vi "DypnlIO.vi"(0 "CMDQueue":refnum<queue>) -> ()   [LabVIEW 2019]
uses:
  <vilib>/Utility/miscctls.llb/LVPointTypeDef.ctl
  <vilib>/Utility/miscctls.llb/LVRectTypeDef.ctl
  SubVIs/ControlProperty.ctl
  user32.dll
panel:
  in  "Boolean":bool
  in  "error in (no error)":errorcluster
  out "error out":errorcluster
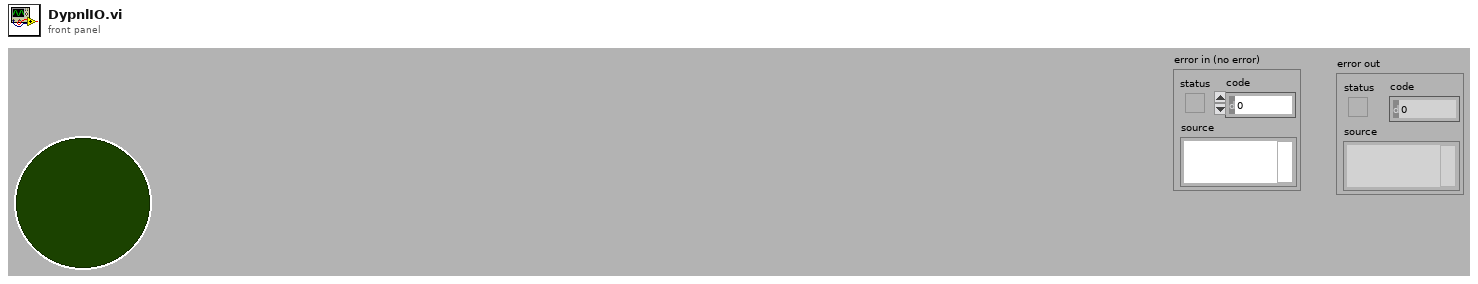
[diagram p1: front panel]
types:
  T1 = enum8{"Enabled", "Disabled", "Disabled and Grayed Out"}
  T2 = typedef "LVPointTypeDef.ctl" = cluster{"Horizontal":i16, "Vertical":i16}
  T3 = typedef "ControlProperty.ctl" = cluster{"Name":string, "WinBounds":T4, "Color":u32, "ShowLabel":bool, "Row/Col":cluster{"Row":u32, "Cols":u32}, "Config":string}
  T4 = typedef "LVRectTypeDef.ctl" = cluster{"Left":i16, "Top":i16, "Right":i16, "Bottom":i16}
  T5 = cluster{"CMD":string, "Parameter":string, "ReturnQueue":refnum<queue>}
  T6 = cluster{"Left":bool, "Top":bool, "Right":bool, "Bottom":bool}
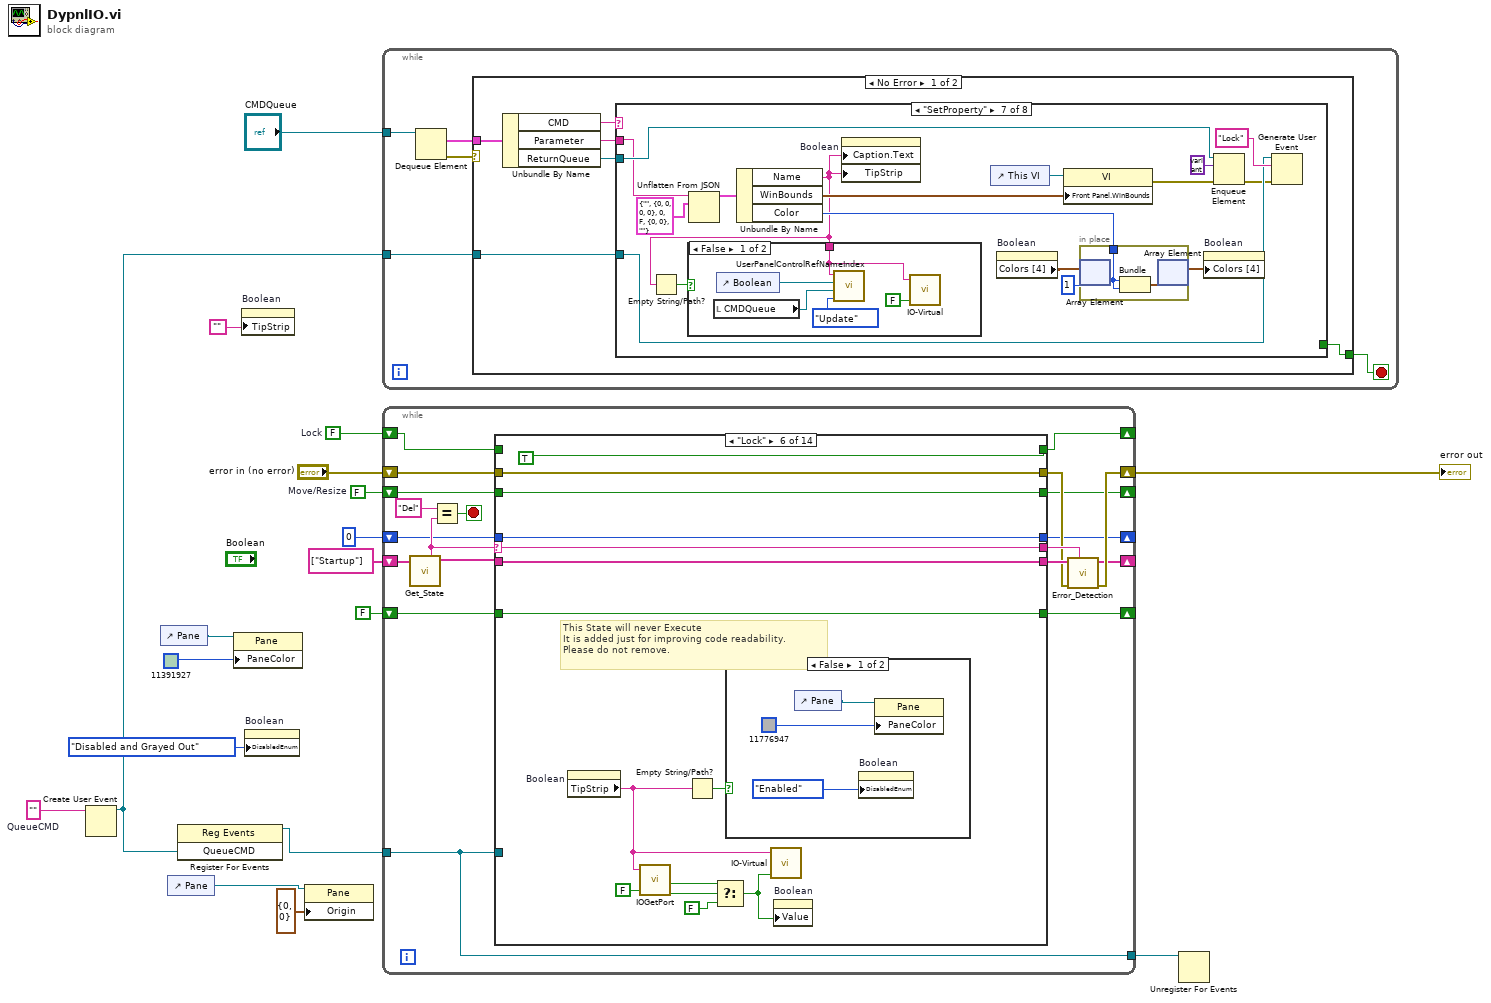
[diagram p0: block diagram]
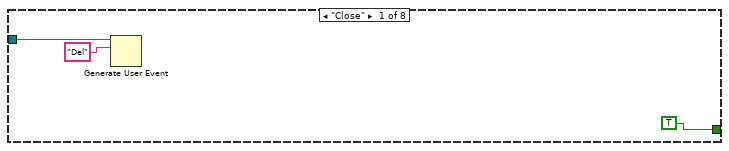
[diagram p2: hidden frame]
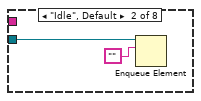
[diagram p3: hidden frame]
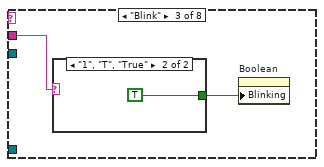
[diagram p4: hidden frame]
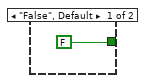
[diagram p5: hidden frame]
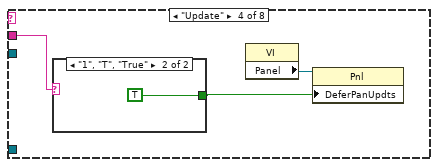
[diagram p6: hidden frame]
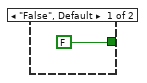
[diagram p7: hidden frame]
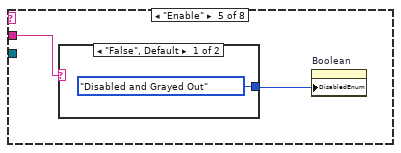
[diagram p8: hidden frame]
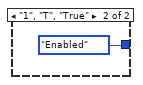
[diagram p9: hidden frame]
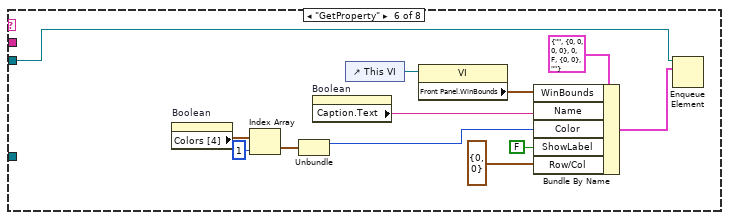
[diagram p10: hidden frame]
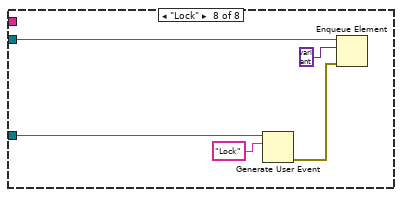
[diagram p12: hidden frame]
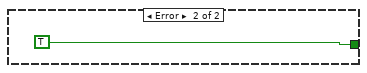
[diagram p13: hidden frame]
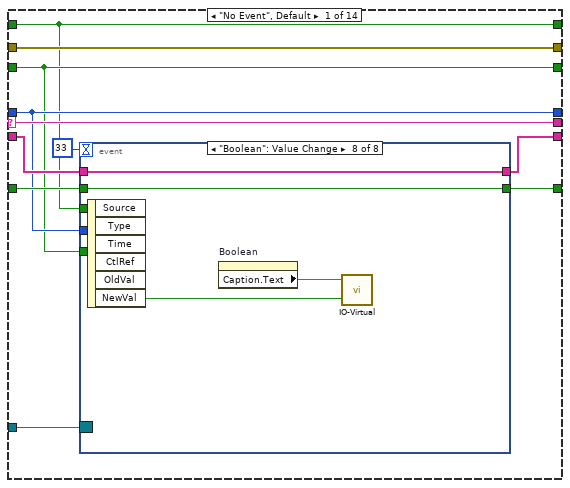
[diagram p14: hidden frame]
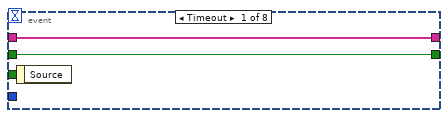
[diagram p15: hidden frame]
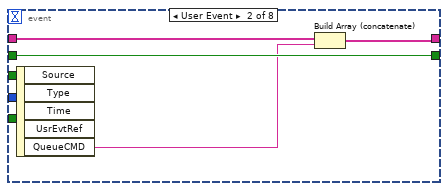
[diagram p16: hidden frame]
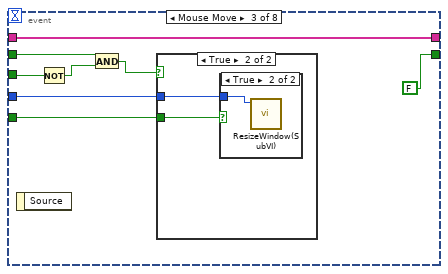
[diagram p17: hidden frame]
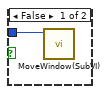
[diagram p19: hidden frame]
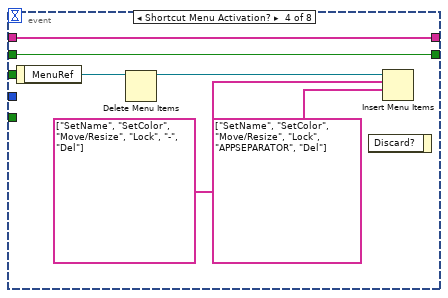
[diagram p20: hidden frame]
diagram:
  w2 = FALSE  # Lock
  w9 = ""  # QueueCMD
  w13 = FALSE  # Move/Resize
  n1 = Create User Event(user event datatype=w9) -> (user event=w6:refnum<user-event>)  [unwired: 1 in, 1 out]
  n2 = control-ref of="Pane"() -> (w4:refnum<vi>)
  n3 = control-ref of="Pane"() -> (w12:refnum<vi>)
  n4 = register-events(w6) -> (reference out=w8:refnum<event-registration>)  [unwired: 2 in, 1 out]
  n5 = property class="Pane"(reference=w4, "PaneColor"=u32 11391927 ("Color Box")) -> ()  [unwired: 1 in, 2 out]
  n6 = property on="Boolean" class="Bool (strict)"("TipStrip"="") -> ()  [unwired: 2 in, 2 out]
  n7 = property on="Boolean" class="Bool (strict)"("DisabledEnum"=T1."Disabled and Grayed Out" ("Disabled")) -> ()  [unwired: 2 in, 2 out]
  n8 = property class="Pane"(reference=w12, "Origin"=T2 {"Horizontal"=0, "Vertical"=0}) -> ()  [unwired: 1 in, 2 out]
  n9 = while {
    tunnel: "CMDQueue" -> [w23]
    tunnel: w6 -> [w19]
    stop <- w21 stop-if-true
    n10 = Dequeue Element(queue=w23) -> (element=w20:T5, error out=w22:errorcluster)  [unwired: 2 in, 2 out]
    n11 = case shown="No Error" w22 {
      tunnel: [w25 TRUE] -> w21
      tunnel: w20 -> [w29 _]
      tunnel: w19 -> [w24 _]
      frame No Error {
        n12 = Unbundle By Name(w29) -> ("CMD"=w28:string, "Parameter"=w26:string, "ReturnQueue"=w27:refnum<queue>)
        n13 = case shown="\"SetProperty\"" w28 {
          tunnel: w27 -> [_ w34 _ _ _ w59 w76 w85]
          tunnel: w26 -> [_ _ w36 w41 w45 _ w71 _]
          tunnel: [TRUE _ _ _ _ _ _ _] -> w25
          tunnel: w24 -> [w31 _ _ _ _ _ w63 w84]
          frame "Close" {
            n14 = Generate User Event(user event=w31, event data cluster="Del" ("event data")) -> ()  [unwired: 2 in, 2 out]
          }
          frame "Idle", Default {
            n15 = Enqueue Element(queue=w34, element="") -> ()  [unwired: 2 in, 3 out]
          }
          frame "Blink" {
            n16 = case shown="\"1\", \"T\", \"True\"" w36 {
              tunnel: [FALSE TRUE] -> w35
              frame "False", Default {
              }
              frame "1", "T", "True" {
              }
            }
            n17 = property on="Boolean" class="Bool (strict)"("Blinking"=w35) -> ()  [unwired: 2 in, 2 out]
          }
          frame "Update" {
            n18 = case shown="\"1\", \"T\", \"True\"" w41 {
              tunnel: [FALSE TRUE] -> w39
              frame "False", Default {
              }
              frame "1", "T", "True" {
              }
            }
            n19 = property class="VI"() -> ("Panel"=w40:refnum<vi>)  [unwired: 2 in, 2 out]
            n20 = property class="Pnl"(reference=w40, "DeferPanUpdts"=w39) -> ()  [unwired: 1 in, 2 out]
          }
          frame "Enable" {
            n21 = case shown="\"False\", Default" w45 {
              tunnel: [T1."Disabled and Grayed Out" ("Disabled") T1."Enabled" ("Disabled")] -> w44
              frame "False", Default {
              }
              frame "1", "T", "True" {
              }
            }
            n22 = property on="Boolean" class="Bool (strict)"("DisabledEnum"=w44) -> ()  [unwired: 2 in, 2 out]
          }
          frame "GetProperty" {
            n23 = property on="Boolean" class="Bool (strict)"() -> ("Colors [4]"=w55:cluster{u32, u32}[])  [unwired: 2 in, 2 out]
            n24 = Index Array(array=w55, index=1) -> (element=w53:cluster{u32, u32})
            n25 = Unbundle(w53) -> (w52:u32)  [unwired: 1 out]
            n26 = property on="Boolean" class="Bool (strict)"() -> ("Caption.Text"=w56:string)  [unwired: 2 in, 2 out]
            n27 = control-ref of="This VI"() -> (w58:refnum<vi>)
            n28 = property class="VI"(reference=w58) -> ("Front Panel.WinBounds"=w57:T4)  [unwired: 1 in, 2 out]
            n29 = Bundle By Name(cluster=T3 {"Name"="", "WinBounds"={"Left"=0, "Top"=0, "Right"=0, "Bottom"=0}, "Color"=0, "ShowLabel"=FALSE, "Row/Col"={"Row"=0, "Cols"=0}, "Config"=""} ("Data"), "WinBounds"=w57, "Name"=w56, "Color"=w52, "ShowLabel"=FALSE, "Row/Col"=cluster{"Row":u32, "Cols":u32} {"Row"=0, "Cols"=0}) -> (w49:T3)
            n30 = Enqueue Element(queue=w59, element=w49) -> ()  [unwired: 2 in, 3 out]
          }
          frame "SetProperty" {
            n31 = Unflatten From JSON(JSON string=w71, type and defaults=T3 {"Name"="", "WinBounds"={"Left"=0, "Top"=0, "Right"=0, "Bottom"=0}, "Color"=0, "ShowLabel"=FALSE, "Row/Col"={"Row"=0, "Cols"=0}, "Config"=""} ("Data")) -> (value=w73:T3)  [unwired: 5 in, 1 out]
            n32 = Unbundle By Name(w73) -> ("Name"=w60:string, "WinBounds"=w70:T4, "Color"=w67:u32)
            n33 = Empty String/Path?(string/path=w60) -> (empty?=w61:bool)
            n34 = case shown="False" w61 {
              tunnel: w60 -> [w77 _]
              frame False {
                n35 = local read "CMDQueue"() -> (w80:refnum<queue>)
                n36 = control-ref of="Boolean"() -> (w79:refnum<vi>)
                n37 = call "UserPanelControlRefNameIndex.vi"("OP"=enum16{"Get", "Update", "Init"}."Update", "CMDQueue"=w80, "UserPanelControlRef"=w79, "ControlName"=w77) -> ()  [unwired: 4 in, 4 out]
                n38 = call "IO-Virtual.vi"("IO"=FALSE, "PortName"=w77) -> ()  [unwired: 3 in, 1 out]
              }
              frame True {
              }
            }
            n39 = property on="Boolean" class="Bool (strict)"("Caption.Text"=w60, "TipStrip"=w60) -> ()  [unwired: 2 in, 2 out]
            n40 = control-ref of="This VI"() -> (w75:refnum<vi>)
            n41 = property on="Boolean" class="Bool (strict)"() -> ("Colors [4]"=w68:cluster{u32, u32}[])  [unwired: 2 in, 2 out]
            n42 = property class="VI"(reference=w75, "Front Panel.WinBounds"=w70) -> (error out=w65:errorcluster)  [unwired: 1 in, 1 out]
            n43 = in-place {
              in-place-border: w67 -> [w82]
              n44 = in-place-array #1(w68, 1) -> ()  [unwired: 1 out]
              n45 = Bundle("Color"=w82, "Color"=w82) -> (w83:cluster{"Color":u32, "Color":u32})  [unwired: 1 in]
              n46 = in-place-array #1(w83) -> (w66:cluster{u32, u32}[])  [unwired: 1 out]
            }
            n47 = property on="Boolean" class="Bool (strict)"("Colors [4]"=w66) -> ()  [unwired: 2 in, 2 out]
            n48 = Enqueue Element(queue=w76, element=variant, error in (no error)=w65) -> (error out=w62:errorcluster)  [unwired: 1 in, 2 out]
            n49 = Generate User Event(user event=w63, event data cluster="Lock" ("event data"), error in=w62) -> ()  [unwired: 1 in, 2 out]
          }
          frame "Lock" {
            n50 = Generate User Event(user event=w84, event data cluster="Lock" ("event data")) -> (error out=w86:errorcluster)  [unwired: 2 in, 1 out]
            n51 = Enqueue Element(queue=w85, element=variant, error in (no error)=w86) -> ()  [unwired: 1 in, 3 out]
          }
        }
      }
      frame Error {
      }
    }
  }
  n52 = while {
    shift-right: [w102] -> _
    shift-left: string[] ["Startup"] ("State Array Out") -> [w101]
    shift-right: [w103] -> w18
    shift-left: "error in (no error)" -> [w107]
    shift-right: [w98] -> _
    shift-left: FALSE -> [w97]
    shift-right: [w96] -> _
    shift-left: u32 0 ("hWnd") -> [w95]
    shift-right: [w94] -> _
    shift-left: w13 -> [w93]
    tunnel: w8 -> [w92]
    tunnel: [w92] -> w7
    shift-right: [w90] -> _
    shift-left: w2 -> [w91]
    stop <- w108 stop-if-true
    n53 = call "Get_State.vi"("State Array In"=w101) -> ("State Array Out"=w100:string[], "Current State"=w99:string)  [unwired: 9 in]
    n54 = Equal?(x="Del", y=w99) -> (x = y?=w108:bool)
    n55 = case shown="\"Lock\"" w99 {
      selector: w99 -> [w120 w186 w192 w199 w212 w226 w240 w256 w271 w278 w285 w293 w311 w323]
      tunnel: w100 -> [w119 w185 w193 w200 w213 w227 w241 w257 w272 w279 w286 w292 w298 w322]
      tunnel: [w116 w184 w193 w200 w213 w227 w241 w257 w272 w279 w286 w292 w298 w322] -> w105
      tunnel: [w117 w182 w191 w198 w211 w225 w239 w255 w270 w277 w284 w291 errorcluster {"status"=FALSE, "code"=0, "source"=""} ("error in (no error)") w319] -> w104
      tunnel: [w120 w186 w192 w199 w212 w226 w240 w256 w271 w278 w285 w293 w311 w323] -> w106
      tunnel: w107 -> [w117 w182 w191 w198 w211 w225 w239 w255 w270 w277 w284 w291 w299 w320]
      tunnel: [w115 w181 w190 w197 w208 w223 w237 w254 w269 w276 w283 w290 w297 w321] -> w98
      tunnel: w97 -> [w114 w181 w190 w197 w208 w223 w237 w254 w269 w276 w283 w290 w297 w321]
      tunnel: [w113 w178 w189 w196 w210 w224 w238 w253 w268 w275 w282 w289 w296 w318] -> w96
      tunnel: w95 -> [w113 _ w189 w196 w210 w224 w238 w253 w268 w275 w282 w289 w296 w318]
      tunnel: w93 -> [w112 w177 w188 w195 w209 w221 w236 w252 w267 w274 w281 w288 w295 w317]
      tunnel: [w112 w177 w188 w195 w207 w221 w236 w252 w267 w274 w281 w288 w295 w317] -> w94
      tunnel: w92 -> [w111 _ _ _ _ _ _ _ _ _ _ _ _ _]
      tunnel: w91 -> [w110 w176 w187 w194 _ _ w231 w251 w266 w273 w280 w287 w294 w316]
      tunnel: [w110 w176 w187 w194 FALSE TRUE w231 w251 w266 w273 w280 w287 w294 w316] -> w90
      frame "No Event", Default {
        n56 = event shown="[7] \"Boolean\": Value Change" {
          selector: w111 -> [_ _ _ _ _ _ _ _]
          dyn-events: _ -> [_ _ _ _ _ _ _ _]
          timeout: 33 -> [_ _ _ _ _ _ _ _]
          tunnel: [w122 w124 w132 w142 w147 w152 w154 w173] -> w116
          tunnel: w119 -> [w122 w125 w132 w142 w147 w153 w155 w173]
          tunnel: [w121 w126 FALSE w139 w146 w150 w156 w172] -> w115
          tunnel: w114 -> [w121 w126 w128 w139 _ w150 w156 w172]
          tunnel: w113 -> [_ _ w133 _ _ _ _ _]
          tunnel: w112 -> [_ _ w131 _ _ _ _ _]
          tunnel: w110 -> [_ _ w129 _ _ _ _ _]
          event Timeout {
            n57 = event-data() -> ()  [unwired: 1 in, 1 out]
          }
          event User Event {
            n58 = event-data() -> ("QueueCMD"=w123:string)  [unwired: 1 in, 4 out]
            n59 = Build Array (concatenate)(w125, w123) -> (w124:string[])
          }
          event Mouse Move {
            n60 = event-data() -> ()  [unwired: 1 in, 1 out]
            n61 = Not(x=w129) -> (.not. x?=w130:bool)
            n62 = And(x=w128, y=w130) -> (x .and. y?=w127:bool)
            n63 = case shown="True" w127 {
              tunnel: w133 -> [_ w136]
              tunnel: w131 -> [_ w135]
              frame False {
              }
              frame True {
                n64 = case shown="True" w135 {
                  tunnel: w136 -> [w137 w138]
                  frame False {
                    n65 = call "MoveWindow(SubVI).vi"("hWnd"=w137) -> ()  [unwired: 10 in, 1 out]
                  }
                  frame True {
                    n66 = call "ResizeWindow(SubVI).vi"("hWnd"=w138) -> ()  [unwired: 10 in, 1 out]
                  }
                }
              }
            }
          }
          event Shortcut Menu Activation? {
            n67 = event-data() -> ("MenuRef"=w141:refnum<k9>)  [unwired: 1 in]
            n68 = Delete Menu Items(9:w141) -> (3:w140:refnum<k9>)  [unwired: 3 in, 1 out]
            n69 = event-data() -> ()  [unwired: 2 in, 1 out]
            n70 = Insert Menu Items(7:string[] ["SetName", "SetColor", "Move/Resize", "Lock", "APPSEPARATOR", "Del"], 8:string[] ["SetName", "SetColor", "Move/Resize", "Lock", "-", "Del"], 9:w140) -> ()  [unwired: 3 in, 3 out]
          }
          event Mouse Down? {
            n71 = event-data() -> ("Button"=w145:u16)  [unwired: 1 in, 1 out]
            n72 = case shown="1" w145 {
              tunnel: [FALSE TRUE] -> w146
              frame 0, Default {
              }
              frame 1 {
              }
            }
            n73 = event-data() -> ()  [unwired: 5 in, 1 out]
          }
          event Shortcut Menu Selection (User) {
            n74 = event-data() -> ("ItemTag"=w151:string)  [unwired: 1 in]
            n75 = Build Array (concatenate)(w153, w151) -> (w152:string[])
          }
          event Panel Resize {
            n76 = event-data() -> ("OldBnds"=w167:T4, "NewBnds"=w166:T4)  [unwired: 1 in, 6 out]
            n77 = Subtract(x=w167, y=w166) -> (x-y=w165:T4)
            n78 = Absolute Value(x=w165) -> (abs(x)=w164:T4)
            n79 = Less?(x=w164, y=T4 {"Left"=3, "Top"=3, "Right"=3, "Bottom"=3}) -> (x < y?=w163:T6)
            n80 = Unbundle(w163) -> ("Left"=w162:bool, "Top"=w161:bool, "Right"=w160:bool, "Bottom"=w159:bool)
            n81 = Compound Arithmetic op=AND(w162, w161, w160, w159) -> (w158:bool)
            n82 = case shown="True" w158 {
              tunnel: w166 -> [_ _]
              tunnel: w155 -> [w168 w171]
              tunnel: [w168 w169] -> w154
              frame False {
              }
              frame True {
                n83 = Build Array (concatenate)(w171, "Redraw" ("event data")) -> (w169:string[])
              }
            }
          }
          event "Boolean": Value Change {
            n84 = event-data() -> ("NewVal"=w175:bool)  [unwired: 1 in, 5 out]
            n85 = property on="Boolean" class="Bool (strict)"() -> ("Caption.Text"=w174:string)  [unwired: 2 in, 2 out]
            n86 = call "IO-Virtual.vi"("IO"=w175, "PortName"=w174) -> ()  [unwired: 3 in, 1 out]
          }
        }
      }
      frame "Startup" {
        # "Get Window Handle"
        n87 = property class="VI"() -> ("Front Panel.Title"=w179:string)  [unwired: 2 in, 2 out]
        n88 = Build Array (concatenate)(w185, string[] [] ("State Array Out")) -> (w184:string[])
        n89 = dll-call lib="user32.dll" fn="FindWindowA"("arg1"=0, "arg2"=w179) -> ("return type"=w178:u32)  [unwired: 5 in, 2 out]
      }
      frame "---------------UI Events---------------" {
        # "This State will never Execute\nIt is added just for improving code readability.\nPlease do not remove."
      }
      frame "---------------Menu Events---------------" {
        # "This State will never Execute\nIt is added just for improving code readability.\nPlease do not remove."
      }
      frame "Move/Resize" {
        # "This State will never Execute\nIt is added just for improving code readability.\nPlease do not remove."
        n90 = Not(x=w209) -> (.not. x?=w207:bool)
        n91 = Select(t=u32 11121611 ("Color Box"), s=w207, f=u32 11391927 ("Color Box")) -> (s? t:f=w205:u32)
        n92 = control-ref of="Pane"() -> (w202:refnum<vi>)
        n93 = property on="Boolean" class="Bool (strict)"("DisabledEnum"=T1."Disabled and Grayed Out" ("Disabled")) -> ()  [unwired: 2 in, 2 out]
        n94 = property class="Pane"(reference=w202, "PaneColor"=w205) -> ()  [unwired: 1 in, 2 out]
      }
      frame "Lock" {
        # "This State will never Execute\nIt is added just for improving code readability.\nPlease do not remove."
        n95 = property on="Boolean" class="Bool (strict)"() -> ("TipStrip"=w215:string)  [unwired: 2 in, 2 out]
        n96 = call "IOGetPort.vi"("Init?"=FALSE, "PortName"=w215) -> ("Find?"=w218:bool, "IO"=w216:bool)  [unwired: 2 in]
        n97 = Empty String/Path?(string/path=w215) -> (empty?=w220:bool)
        n98 = Select(t=w216, s=w218, f=FALSE) -> (s? t:f=w214:bool)
        n99 = case shown="False" w220 {
          frame False {
            n100 = control-ref of="Pane"() -> (w230:refnum<vi>)
            n101 = property on="Boolean" class="Bool (strict)"("DisabledEnum"=T1."Enabled" ("Disabled")) -> ()  [unwired: 2 in, 2 out]
            n102 = property class="Pane"(reference=w230, "PaneColor"=u32 11776947 ("Color Box")) -> ()  [unwired: 1 in, 2 out]
          }
          frame True {
          }
        }
        n103 = call "IO-Virtual.vi"("IO"=w214, "PortName"=w215) -> ()  [unwired: 3 in, 1 out]
        n104 = property on="Boolean" class="Bool (strict)"("Value"=w214) -> ()  [unwired: 2 in, 2 out]
      }
      frame "SetColor" {
        # "This State will never Execute\nIt is added just for improving code readability.\nPlease do not remove."
        n105 = call "DyanmicPanelControlColor.vi"() -> ("ColorOut"=w233:u32)
        n106 = property on="Boolean" class="Bool (strict)"() -> ("Colors [4]"=w235:cluster{u32, u32}[])  [unwired: 2 in, 2 out]
        n107 = in-place {
          in-place-border: w233 -> [w243]
          n108 = in-place-array #2(w235, 1) -> ()  [unwired: 1 out]
          n109 = Bundle("ColorOut"=w243, "ColorOut"=w243) -> (w242:cluster{"ColorOut":u32, "ColorOut":u32})  [unwired: 1 in]
          n110 = in-place-array #2(w242) -> (w232:cluster{u32, u32}[])  [unwired: 1 out]
        }
        n111 = property on="Boolean" class="Bool (strict)"("Colors [4]"=w232) -> ()  [unwired: 2 in, 2 out]
      }
      frame "SetName" {
        # "This State will never Execute\nIt is added just for improving code readability.\nPlease do not remove."
        n112 = property on="Boolean" class="Bool (strict)"() -> ("TipStrip"=w247:string)  [unwired: 2 in, 2 out]
        n113 = Empty String/Path?(string/path=w247) -> (empty?=w248:bool)
        n114 = Select(t="IO" ("f"), s=w248, f=w247) -> (s? t:f=w249:string)
        n115 = call "DyanmicPanelControlSetName.vi"("ControlNameIn"=w249) -> ("ControlName"=w250:string, "Find?"=w245:bool)  [unwired: 1 in]
        n116 = case shown="True" w245 {
          tunnel: [TRUE ("T button?") w259] -> w244
          frame False {
          }
          frame True {
            n117 = Two Button Dialog(message="Control Name exits, Confirm to Over Write?") -> (T button?=w259:bool)  [unwired: 2 in]
          }
        }
        n118 = case shown="True" w244 {
          tunnel: w250 -> [_ w261]
          frame False {
          }
          frame True {
            n119 = local read "CMDQueue"() -> (w264:refnum<queue>)
            n120 = control-ref of="Boolean"() -> (w265:refnum<vi>)
            n121 = property on="Boolean" class="Bool (strict)"("TipStrip"=w261, "Caption.Text"=w261) -> ()  [unwired: 2 in, 2 out]
            n122 = call "UserPanelControlRefNameIndex.vi"("OP"=enum16{"Get", "Update", "Init"}."Update", "CMDQueue"=w264, "UserPanelControlRef"=w265, "ControlName"=w261) -> ()  [unwired: 4 in, 4 out]
            n123 = call "IO-Virtual.vi"("IO"=FALSE, "PortName"=w261) -> ()  [unwired: 3 in, 1 out]
          }
        }
      }
      frame "Redraw" {
        # "This State will never Execute\nIt is added just for improving code readability.\nPlease do not remove."
      }
      frame "---------------Client Events---------------" {
        # "This State will never Execute\nIt is added just for improving code readability.\nPlease do not remove."
      }
      frame "---------------Subroutine states---------------" {
        # "This State will never Execute\nIt is added just for improving code readability.\nPlease do not remove."
      }
      frame "---------------Error Handling VIs---------------" {
        # "This State will never Execute\nIt is added just for improving code readability.\nPlease do not remove."
      }
      frame "Error" {
        n124 = Call Chain() -> (call chain=w306:string[])
        n125 = for {
          tunnel: w306 -> [w314] mode=indexing
          shift-right: [w312] -> w303
          shift-left: "" -> [w315]
          n126 = Concatenate Strings(w315, w314, " -> ") -> (w312:string)
        }
        n127 = Unbundle By Name(w299) -> ("code"=w301:i32, "source"=w300:string)
        n128 = Match Pattern(string=w300, regular expression=":") -> (before substring=w304:string, after substring=w308:string)  [unwired: 1 in, 2 out]
        n129 = Format Into String(format string="Error Occured In\"%s\" state of \"%s\" VI\nError Code: %d\nError Description: \"%s\"", w304, w303, w301, w308) -> (resulting string=w307:string)  [unwired: 2 in, 1 out]
        n130 = One Button Dialog(message=w307) -> ()  [unwired: 1 in, 1 out]
      }
      frame "Del", "Exit" {
        n131 = invoke class="VI" method="FP.Close"(error in=w320) -> (error out=w319:errorcluster)  [unwired: 2 in, 2 out]
      }
    }
    n132 = call "Error_Detection.vi"("Current State"=w106, "error in (no error)"=w104, "Msg In"=w105) -> ("error out"=w103:errorcluster, "Msg Out"=w102:string[])  [unwired: 7 in]
  }
  "error out" <- w18
  n133 = Unregister For Events(event registration refnum=w7) -> ()  [unwired: 1 in, 1 out]
